vi "RegisteredMessages.vi"() -> (3 "registered messages":string[](array[string]))   [LabVIEW 2017, in "IrManageCameras.lvlib"]
uses:
  <vilib>/addons/InsightCM/Devices/Shared/Ir/IrManageCameras/IrManageCameras.lvlib
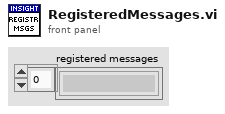
[diagram p1: front panel]
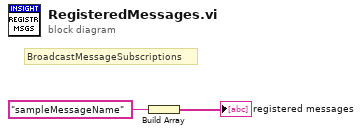
[diagram p0: block diagram]
diagram:
  # "BroadcastMessageSubscriptions"
  n1 = Build Array("sampleMessageName" ("String")) -> (→"registered messages":string[])
